vi "Connected.vi"(8 "error in (no error)":errorcluster, 9 "Message Stream":refnum<class "Message Stream.lvclass">, 10 "Endpoint Enqueuer":refnum<class "Message Enqueuer.lvclass">, 11 "Server in":refnum<class "Server.lvclass">) -> (0 "error out":errorcluster, 3 "Server out":refnum<class "Server.lvclass">)   [LabVIEW 2021, in "Server.lvlib" / "Server.lvclass"]
uses:
  Server.lvclass
  <vilib>/ActorFramework/Message Enqueuer/Message Enqueuer.lvclass
  <vilib>/NI/Actors/Network Endpoint Actors/Abstract Classes/Message Stream/Message Stream.lvclass
  Server.lvclass/Server.ctl
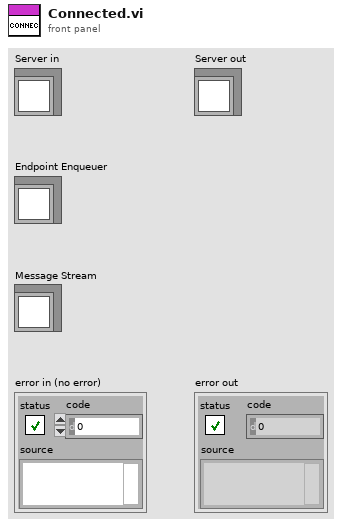
[diagram p1: front panel]
types:
  T1 = enum8{"Enabled", "Disabled", "Disabled and Grayed Out"}
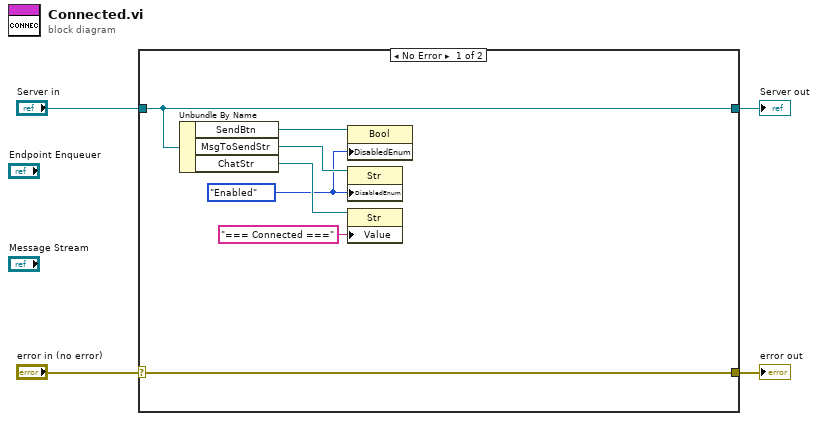
[diagram p0: block diagram]
diagram:
  n1 = case shown="No Error" "error in (no error)" {
    selector: "error in (no error)" -> [w11 w13]
    tunnel: [w11 w13] -> w3
    tunnel: [w10 w12] -> w1
    tunnel: "Server in" -> [w10 w12]
    frame No Error {
      w6 = T1."Enabled" ("Disabled")
      n2 = Unbundle By Name(w10) -> ("SendBtn"=w9:refnum<vi>, "MsgToSendStr"=w8:refnum<vi>, "ChatStr"=w7:refnum<vi>)
      n3 = property class="Bool"(reference=w9, "DisabledEnum"=w6) -> ()  [unwired: 1 in, 2 out]
      n4 = property class="Str"(reference=w8, "DisabledEnum"=w6) -> ()  [unwired: 1 in, 2 out]
      n5 = property class="Str"(reference=w7, "Value"="=== Connected ===") -> ()  [unwired: 1 in, 2 out]
    }
    frame Error {
    }
  }
  "error out" <- w3
  "Server out" <- w1
